vi "S2C_M2p5942_Proc_Acquisition.vi"(7 "Local?":bool, 8 "Error In":errorcluster, 10 "Command":string, 11 "JSON String":string) -> (0 "Error Out":errorcluster, 3 "Response":variant)   [LabVIEW 2024]
uses:
  S2C_M2p5942_Proc_Globals.vi
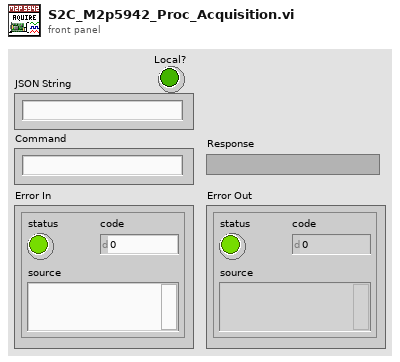
[diagram p1: front panel]
types:
  T1 = cluster{"Single Shot":bool, "Loop":bool, "Force Trigger":bool, "Status":string, "Stop":bool}
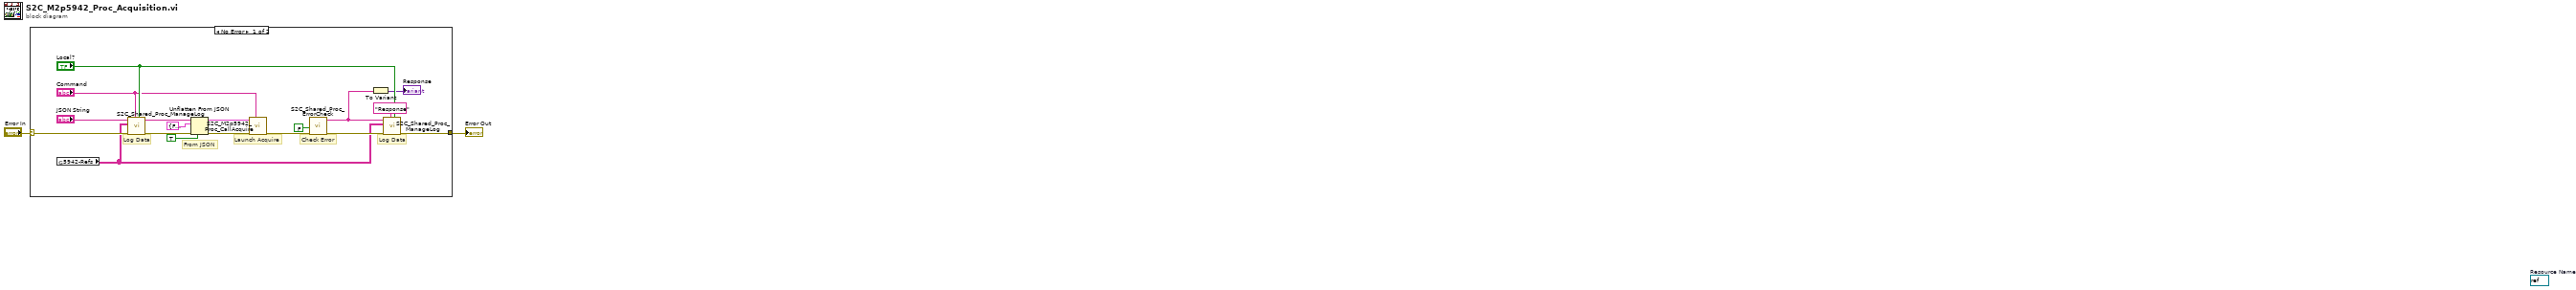
[diagram p0: block diagram]
diagram:
  (unwired) refnum<visa-resource-name> refnum  # Resource Name
  n1 = case shown="No Error" "Error In" {
    selector: "Error In" -> [w19 w21]
    tunnel: [w17 w21] -> w1
    frame No Error {
      # "Launch Acquire"
      # "Check Error"
      # "Log Data"
      # "Log Data"
      # "From JSON"
      n2 = global read "S2C_M2p5942_Proc_Globals.vi" "5942-Refs"() -> (w12:string[][])
      n3 = call "S2C_Shared_Proc_ManageLog.vi"("Local?"="Local?", "Command"="Command", "Error In"=w19, "Refs"=w12, "Data In"="JSON String") -> ("Error Out"=w9:errorcluster, "Data Out"=w8:string)  [unwired: 5 in]
      n4 = Unflatten From JSON(JSON string=w8, type and defaults=T1 {"Single Shot"=FALSE, "Loop"=FALSE, "Force Trigger"=FALSE, "Status"="", "Stop"=FALSE} ("Acquisition"), default null elements? (F)=TRUE, error in (no error)=w9) -> (value=w5:T1, error out=w7:errorcluster)  [unwired: 3 in]
      n5 = call "S2C_M2p5942_Proc_CallAcquire.vi"("Command"="Command", "Error In"=w7, "Data"=w5) -> ("Error Out"=w4:errorcluster)  [unwired: 8 in]
      n6 = call "S2C_Shared_Proc_ErrorCheck.vi"("Error In"=w4, "ExpReply?"=FALSE) -> ("Error Out"=w14:errorcluster, "Status"=w11:string)  [unwired: 8 in]
      n7 = To Variant(anything=w11) -> (Variant=→"Response":variant)
      n8 = call "S2C_Shared_Proc_ManageLog.vi"("Local?"="Local?", "Command"="Response", "Error In"=w14, "Refs"=w12, "Data In"=w11) -> ("Error Out"=w17:errorcluster)  [unwired: 5 in, 1 out]
    }
    frame Error {
    }
  }
  "Error Out" <- w1
